vi "Tools_System Drive Status.vi"(8 "error in (no error)":errorcluster, 11 "Drive":path=path "c:/") -> (0 "error out":errorcluster, 1 "Free drive space (%)":dbl, 2 "Free drive space (GB)":dbl, 3 "Drive size (GB)":dbl)   [LabVIEW 2009]
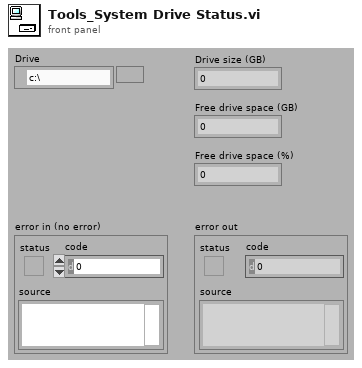
[diagram p1: front panel]
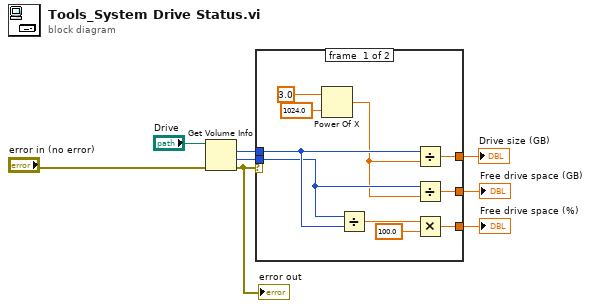
[diagram p0: block diagram]
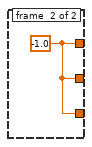
[diagram p2: hidden frame]
diagram:
  n1 = Get Volume Info(8:"error in (no error)", 11:"Drive") -> (0:w1:errorcluster, 1:w4:i64, 2:w3:i64)  [unwired: 3 out]
  "error out" <- w1
  n2 = case shown="No Error" w1 {
    tunnel: [w16 w19] -> w7
    tunnel: w3 -> [w13 _]
    tunnel: w4 -> [w12 _]
    tunnel: [w10 w19] -> w5
    tunnel: [w9 w19] -> w6
    frame #0 {
      n3 = Power Of X(1:1024.0 ("x"), 2:3.0 ("y")) -> (0:w11:dbl)
      n4 = Divide(x=w12, y=w13) -> (x/y=w18:dbl)
      n5 = Divide(x=w13, y=w11) -> (x/y=w10:dbl)
      n6 = Divide(x=w12, y=w11) -> (x/y=w9:dbl)
      n7 = Multiply(x=w18, y=100.0) -> (x*y=w16:dbl)
    }
    frame #1 {
      w19 = -1.0
    }
  }
  "Free drive space (%)" <- w7
  "Free drive space (GB)" <- w6
  "Drive size (GB)" <- w5
